vi "Get Time Trace.vi"(0 "Channel Index":i32) -> (1 "Time (s)":dbl[](array[numeric]), 2 "Time Array index":i32)   [LabVIEW 2022 SP3]
uses:
  Globals/Meas_global.vi
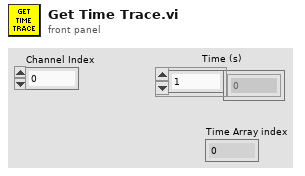
[diagram p1: front panel]
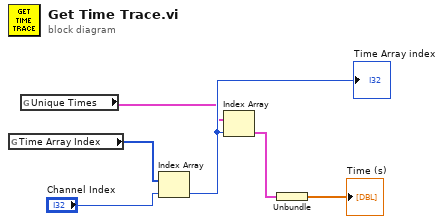
[diagram p0: block diagram]
diagram:
  n1 = global read "Meas_global.vi" "Time Array Index"() -> (w6:i32[])
  n2 = global read "Meas_global.vi" "Unique Times"() -> (w3:cluster{"Time (s)":dbl[]}[])
  n3 = Index Array(array=w6, index="Channel Index") -> (element=w4:i32)
  "Time Array index" <- w4
  n4 = Index Array(array=w3, index=w4) -> (element=w2:cluster{"Time (s)":dbl[]})
  n5 = Unbundle(w2) -> ("Time (s)"=→"Time (s)":dbl[])
